vi "pressmon.vi"() -> ()   [LabVIEW 2015]
panel:
  in  "START":bool
  in  "KILL":bool
  in  "PAUSE":bool
  in  "RESUME":bool
  in  "QUIT":bool
  out "return code":i32
  in  "stop & close prog":bool
  out "standard error":string
  out "standard output":string
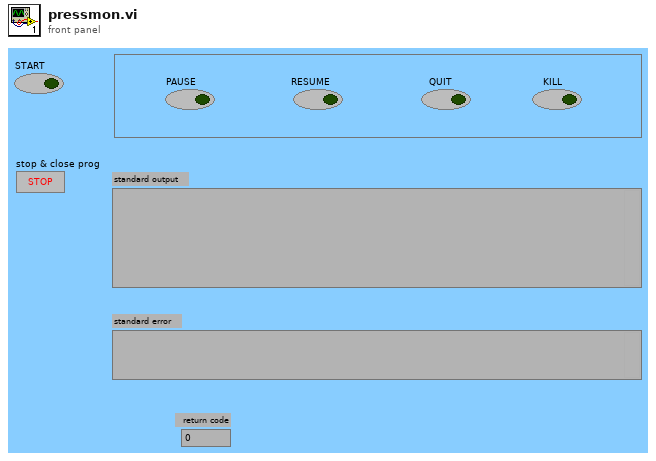
[diagram p1: front panel]
types:
  T1 = enum16{"open", "replace", "create", "open or create", "replace or create", "replace or create with confirmation"}
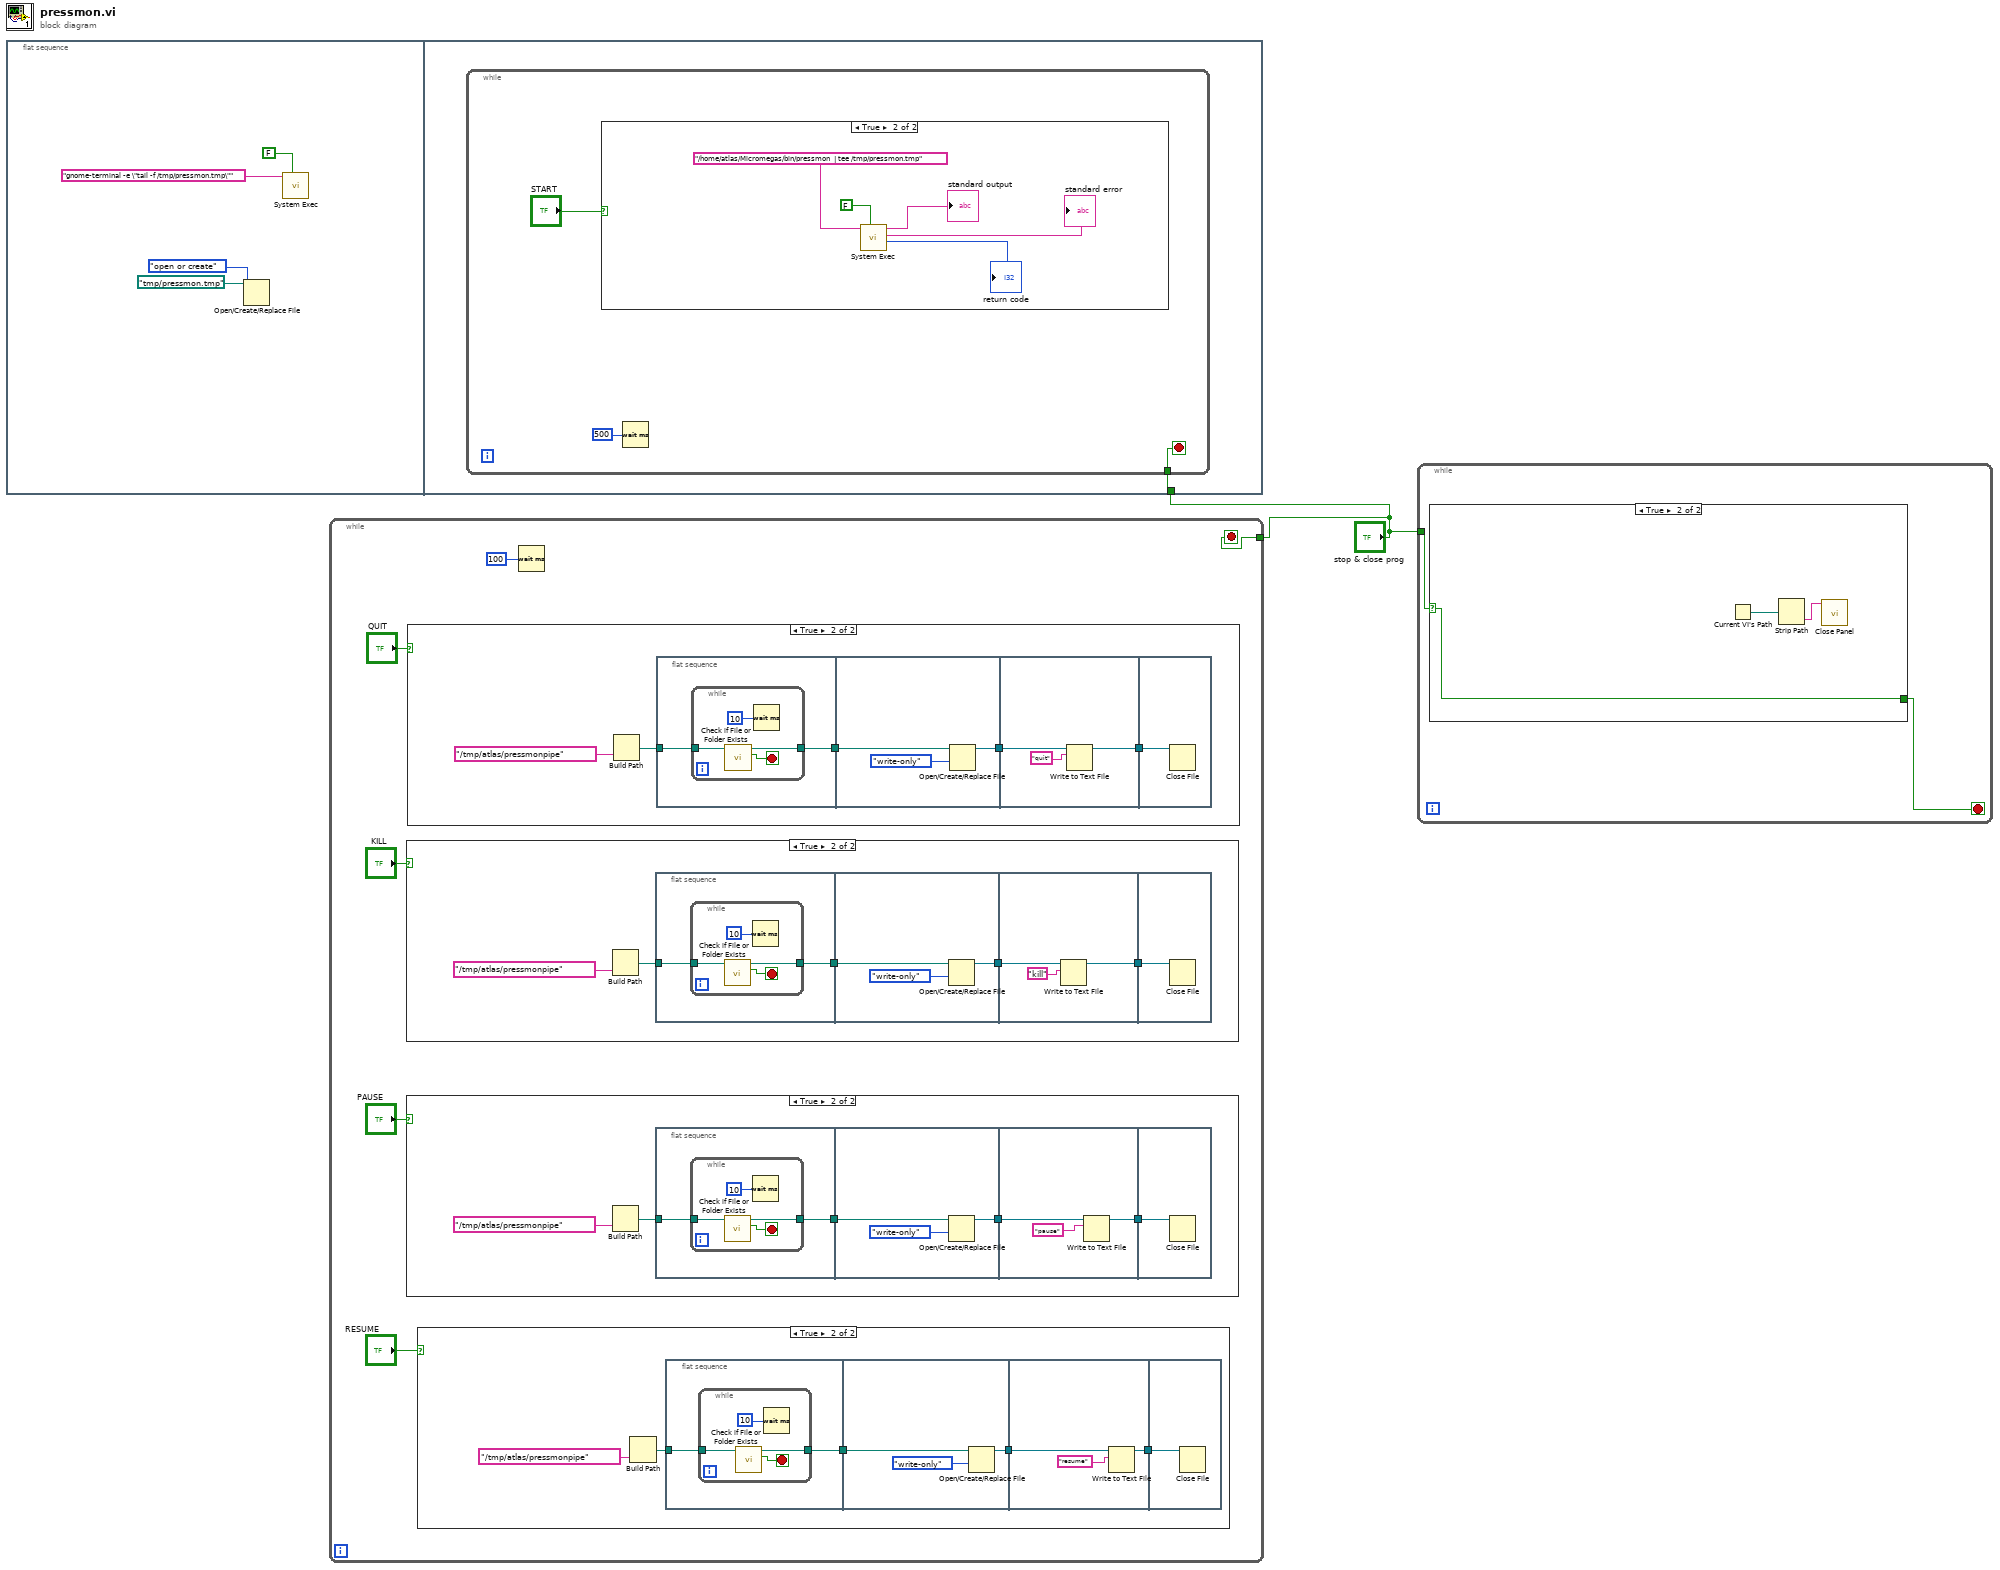
[diagram p0: block diagram]
diagram:
  n1 = flat-sequence {
    tunnel: "stop & close prog" -> [w6]
    frame #0 {
      n2 = Open/Create/Replace File(file path (use dialog)=path "/tmp/pressmon.tmp", operation (0:open)=T1."open or create") -> ()  [unwired: 4 in, 3 out]
      n3 = call <vilib>:"System Exec.vi"("wait until completion? (T)"=FALSE, "command line"="gnome-terminal -e \"tail -f /tmp/pressmon.tmp\"") -> ()  [unwired: 6 in, 4 out]
    }
    frame #1 {
      n4 = while {
        tunnel: w6 -> [w8]
        stop <- w8 stop-if-true
        n5 = case shown="True" "START" {
          frame False {
          }
          frame True {
            n6 = call <vilib>:"System Exec.vi"("wait until completion? (T)"=FALSE, "command line"="/home/atlas/Micromegas/bin/pressmon  | tee /tmp/pressmon.tmp") -> ("return code"=→"return code":i32, "standard error"=→"standard error":string, "standard output"=→"standard output":string)  [unwired: 6 in, 1 out]
          }
        }
        n7 = Wait (ms)(milliseconds to wait=u32 500) -> ()  [unwired: 1 out]
      }
    }
  }
  n8 = while {
    tunnel: "stop & close prog" -> [w15]
    stop <- w15 stop-if-true
    n9 = case shown="True" "KILL" {
      frame False {
      }
      frame True {
        n10 = Build Path(name or relative path="/tmp/atlas/pressmonpipe" ("string")) -> (appended path=w39:path)  [unwired: 1 in]
        n11 = flat-sequence {
          tunnel: [w45] -> w43
          tunnel: w39 -> [w44]
          tunnel: w43 -> [w52]
          tunnel: [w50] -> w42
          tunnel: w42 -> [w55]
          tunnel: [w54] -> w41
          tunnel: w41 -> [w56]
          frame #0 {
            n12 = while {
              tunnel: [w47] -> w45
              tunnel: w44 -> [w46]
              stop <- w48 stop-if-true
              n13 = call <vilib>:"Check if File or Folder Exists.vi"("path"=w46) -> ("file or folder exists?"=w48:bool, "dup path"=w47:path)  [unwired: 8 in, 1 out]
              n14 = Wait (ms)(milliseconds to wait=u32 10) -> ()  [unwired: 1 out]
            }
          }
          frame #1 {
            n15 = Open/Create/Replace File(file path (use dialog)=w52, access (0:read/write)=enum16{"read/write", "read-only", "write-only"}."write-only") -> (refnum out=w50:refnum<file>)  [unwired: 4 in, 2 out]
          }
          frame #2 {
            n16 = Write to Text File(file (use dialog)=w55, text="kill") -> (refnum out=w54:refnum<file>)  [unwired: 2 in, 2 out]
          }
          frame #3 {
            n17 = Close File(refnum=w56) -> ()  [unwired: 1 in, 2 out]
          }
        }
      }
    }
    n18 = case shown="True" "PAUSE" {
      frame False {
      }
      frame True {
        n19 = Build Path(name or relative path="/tmp/atlas/pressmonpipe" ("string")) -> (appended path=w21:path)  [unwired: 1 in]
        n20 = flat-sequence {
          tunnel: [w27] -> w25
          tunnel: w21 -> [w26]
          tunnel: w25 -> [w34]
          tunnel: [w32] -> w24
          tunnel: w24 -> [w37]
          tunnel: [w36] -> w23
          tunnel: w23 -> [w38]
          frame #0 {
            n21 = while {
              tunnel: [w29] -> w27
              tunnel: w26 -> [w28]
              stop <- w30 stop-if-true
              n22 = call <vilib>:"Check if File or Folder Exists.vi"("path"=w28) -> ("file or folder exists?"=w30:bool, "dup path"=w29:path)  [unwired: 8 in, 1 out]
              n23 = Wait (ms)(milliseconds to wait=u32 10) -> ()  [unwired: 1 out]
            }
          }
          frame #1 {
            n24 = Open/Create/Replace File(file path (use dialog)=w34, access (0:read/write)=enum16{"read/write", "read-only", "write-only"}."write-only") -> (refnum out=w32:refnum<file>)  [unwired: 4 in, 2 out]
          }
          frame #2 {
            n25 = Write to Text File(file (use dialog)=w37, text="pause") -> (refnum out=w36:refnum<file>)  [unwired: 2 in, 2 out]
          }
          frame #3 {
            n26 = Close File(refnum=w38) -> ()  [unwired: 1 in, 2 out]
          }
        }
      }
    }
    n27 = case shown="True" "QUIT" {
      frame False {
      }
      frame True {
        n28 = Build Path(name or relative path="/tmp/atlas/pressmonpipe" ("string")) -> (appended path=w75:path)  [unwired: 1 in]
        n29 = flat-sequence {
          tunnel: [w81] -> w79
          tunnel: w75 -> [w80]
          tunnel: w79 -> [w88]
          tunnel: [w86] -> w78
          tunnel: w78 -> [w91]
          tunnel: [w90] -> w77
          tunnel: w77 -> [w92]
          frame #0 {
            n30 = while {
              tunnel: [w83] -> w81
              tunnel: w80 -> [w82]
              stop <- w84 stop-if-true
              n31 = call <vilib>:"Check if File or Folder Exists.vi"("path"=w82) -> ("file or folder exists?"=w84:bool, "dup path"=w83:path)  [unwired: 8 in, 1 out]
              n32 = Wait (ms)(milliseconds to wait=u32 10) -> ()  [unwired: 1 out]
            }
          }
          frame #1 {
            n33 = Open/Create/Replace File(file path (use dialog)=w88, access (0:read/write)=enum16{"read/write", "read-only", "write-only"}."write-only") -> (refnum out=w86:refnum<file>)  [unwired: 4 in, 2 out]
          }
          frame #2 {
            n34 = Write to Text File(file (use dialog)=w91, text="quit") -> (refnum out=w90:refnum<file>)  [unwired: 2 in, 2 out]
          }
          frame #3 {
            n35 = Close File(refnum=w92) -> ()  [unwired: 1 in, 2 out]
          }
        }
      }
    }
    n36 = case shown="True" "RESUME" {
      frame False {
      }
      frame True {
        n37 = Build Path(name or relative path="/tmp/atlas/pressmonpipe" ("string")) -> (appended path=w57:path)  [unwired: 1 in]
        n38 = flat-sequence {
          tunnel: [w63] -> w61
          tunnel: w57 -> [w62]
          tunnel: w61 -> [w70]
          tunnel: [w68] -> w60
          tunnel: w60 -> [w73]
          tunnel: [w72] -> w59
          tunnel: w59 -> [w74]
          frame #0 {
            n39 = while {
              tunnel: [w65] -> w63
              tunnel: w62 -> [w64]
              stop <- w66 stop-if-true
              n40 = call <vilib>:"Check if File or Folder Exists.vi"("path"=w64) -> ("file or folder exists?"=w66:bool, "dup path"=w65:path)  [unwired: 8 in, 1 out]
              n41 = Wait (ms)(milliseconds to wait=u32 10) -> ()  [unwired: 1 out]
            }
          }
          frame #1 {
            n42 = Open/Create/Replace File(file path (use dialog)=w70, access (0:read/write)=enum16{"read/write", "read-only", "write-only"}."write-only") -> (refnum out=w68:refnum<file>)  [unwired: 4 in, 2 out]
          }
          frame #2 {
            n43 = Write to Text File(file (use dialog)=w73, text="resume") -> (refnum out=w72:refnum<file>)  [unwired: 2 in, 2 out]
          }
          frame #3 {
            n44 = Close File(refnum=w74) -> ()  [unwired: 1 in, 2 out]
          }
        }
      }
    }
    n45 = Wait (ms)(milliseconds to wait=100) -> ()  [unwired: 1 out]
  }
  n46 = while {
    tunnel: "stop & close prog" -> [w94]
    stop <- w93 stop-if-true
    n47 = case shown="True" w94 {
      selector: w94 -> [w95 w98]
      tunnel: [w95 w98] -> w93
      frame False {
      }
      frame True {
        n48 = Current VI's Path() -> (path=w96:path)
        n49 = Strip Path(path=w96) -> (name=w97:string)  [unwired: 1 out]
        n50 = call <vilib>:"Close Panel.vi"("VI name"=w97) -> ()  [unwired: 10 in, 1 out]
      }
    }
  }
